vi "Micros read and write v3.vi"() -> ()   [LabVIEW 2017]
uses:
  <vilib>/Instr/_visa.llb/VISA Configure Serial Port (Instr).vi
panel:
  out "Voltaje de salida":dbl[](array[numeric])
  out "Salida de Voltaje":dbl[](graph)
  in  "write buffer":string
  in  "stop":bool
  out "Numero de Bytes":u32
  out "ASCII/Valor de entrada":string
  in  "VISA resource name":refnum<visa-resource-name>
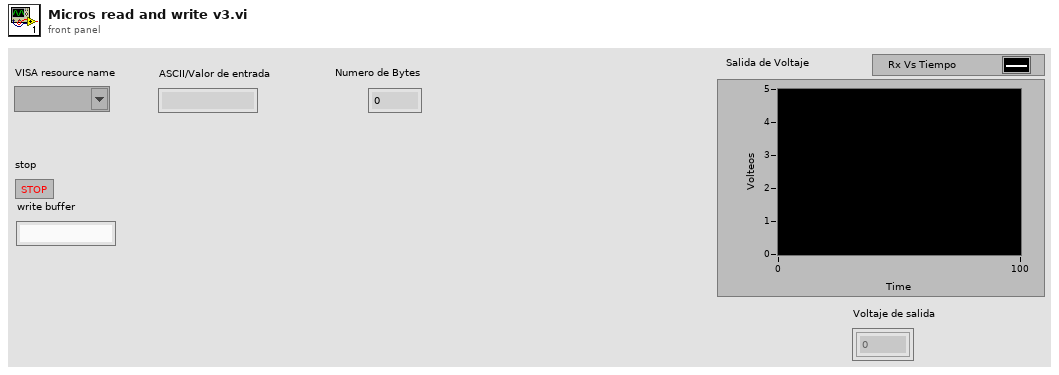
[diagram p1: front panel]
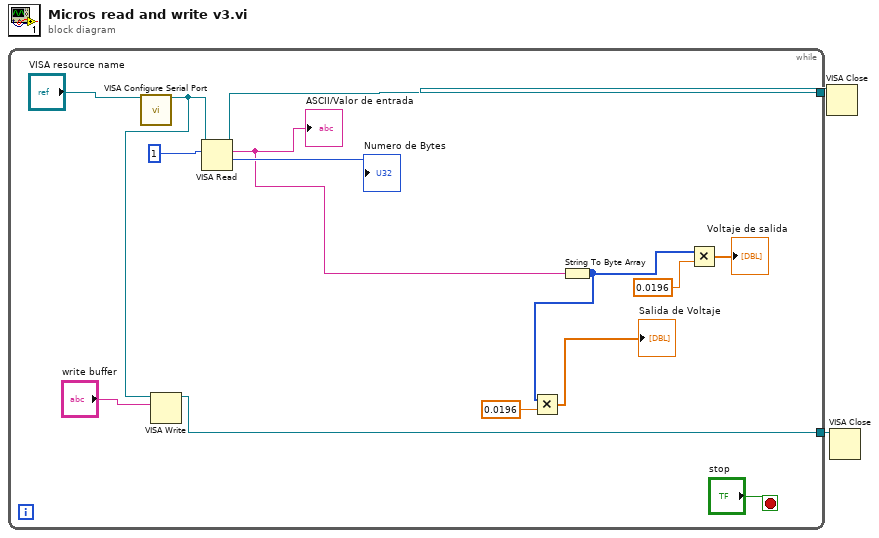
[diagram p0: block diagram]
diagram:
  n1 = while {
    tunnel: [w15] -> w2
    tunnel: [w11] -> w1
    stop <- "stop" stop-if-true
    n2 = call-poly "VISA Configure Serial Port"("VISA resource name"="VISA resource name") -> ("VISA resource name out"=w10:refnum<visa-resource-name>)  [unwired: 13 in, 1 out]
    n3 = VISA Write(VISA resource name=w10, write buffer="write buffer") -> (VISA resource name out=w11:refnum<visa-resource-name>)  [unwired: 1 in, 2 out]
    n4 = VISA Read(VISA resource name=w10, byte count=u32 1) -> (VISA resource name out=w15:refnum<visa-resource-name>, read buffer=w9:string, return count=→"Numero de Bytes":u32)  [unwired: 1 in, 1 out]
    "ASCII/Valor de entrada" <- w9
    n5 = String To Byte Array(string=w9) -> (unsigned byte array=w5:u8[])
    n6 = Multiply(x=w5, y=0.0196) -> (x*y=→"Salida de Voltaje":dbl[])
    n7 = Multiply(x=w5, y=0.0196) -> (x*y=→"Voltaje de salida":dbl[])
  }
  n8 = VISA Close(VISA resource name=w2) -> ()  [unwired: 1 in, 1 out]
  n9 = VISA Close(VISA resource name=w1) -> ()  [unwired: 1 in, 1 out]
